vi "ctiRMShodnoty.vi"(8 "vstupniError":errorcluster, 11 "vstupniNotifier":refnum<notifier>) -> (0 "vystupniError":errorcluster, 2 "RMS filtrovaného signálu":dbl, 3 "RMS original signálu":dbl)   [LabVIEW 2018]
panel:
  # "Vstupy:"
  # "Vystupy:"
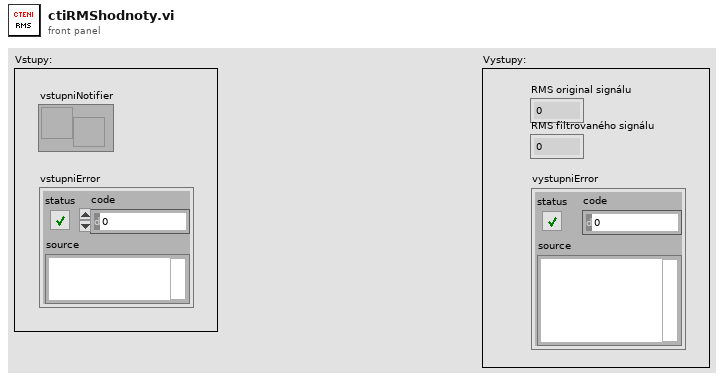
[diagram p1: front panel]
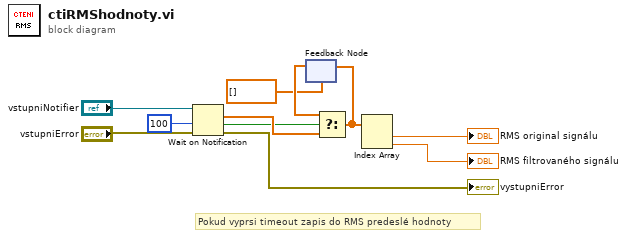
[diagram p0: block diagram]
diagram:
  # "Pokud vyprsi timeout zapis do RMS predeslé hodnoty"
  n1 = Wait on Notification(notifier="vstupniNotifier", timeout in ms (-1)=100, error in (no error)="vstupniError") -> (notification=w9:dbl[], timed out?=w8:bool, error out=→"vystupniError":errorcluster)  [unwired: 1 in, 1 out]
  n2 = feedback #1(dbl[] [] ("s? t:f")) -> (w3:dbl[])
  n3 = Select(t=w3, s=w8, f=w9) -> (s? t:f=w2:dbl[])
  n4 = feedback-in #1(w2) -> ()
  n5 = Index Array(array=w2) -> (element #1=→"RMS original signálu":dbl, element #2=→"RMS filtrovaného signálu":dbl)  [unwired: 2 in]
